vi "Read All Files In Folder.vi"(8 "error in (no error)":errorcluster, 10 "FolderPath":path, 11 "Old File Path":path) -> (0 "error out":errorcluster, 1 "File Name":string, 2 "New File Path":path, 3 "File Paths":path[](array[path]))   [LabVIEW 2020, in "DocTool.lvlib"]
uses:
  DocTool.lvlib
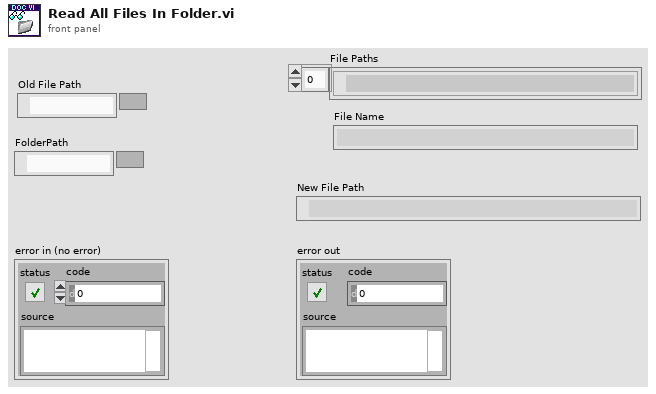
[diagram p1: front panel]
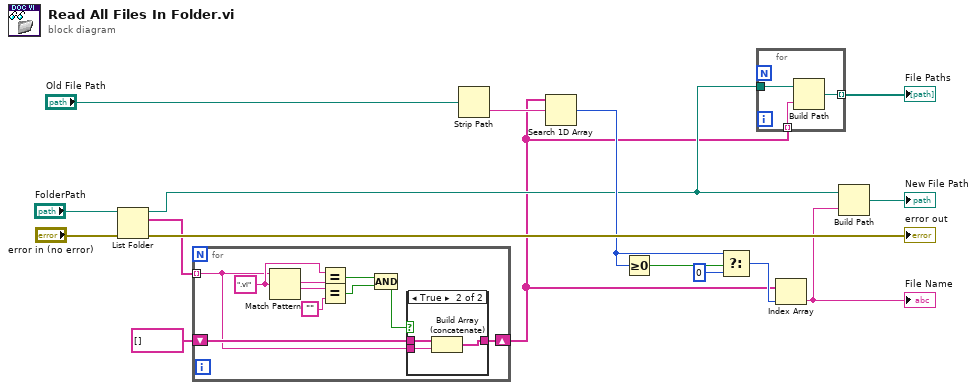
[diagram p0: block diagram]
diagram:
  n1 = List Folder(path="FolderPath", error in="error in (no error)") -> (path out=w5:path, filenames=w4:string[], error out=→"error out":errorcluster)  [unwired: 2 in, 1 out]
  n2 = for {
    tunnel: w4 -> [w20] mode=indexing
    shift-right: [w25] -> w1
    shift-left: string[] [] ("filenames") -> [w26]
    w21 = ".vi" ("string")
    n3 = Match Pattern(string=w20, regular expression=w21) -> (match substring=w22:string, after substring=w24:string)  [unwired: 1 in, 2 out]
    n4 = Equal?(x=w21, y=w22) -> (x = y?=w17:bool)
    n5 = Equal?(x=w24, y="") -> (x = y?=w18:bool)
    n6 = Compound Arithmetic op=AND(w17, w18) -> (w19:bool)
    n7 = case shown="True" w19 {
      tunnel: w26 -> [w27 w30]
      tunnel: [w27 w29] -> w25
      tunnel: w20 -> [_ w28]
      frame False {
      }
      frame True {
        n8 = Build Array (concatenate)(w30, w28) -> (w29:string[])
      }
    }
  }
  n9 = Strip Path(path="Old File Path") -> (name=w10:string)  [unwired: 1 out]
  n10 = Search 1D Array(1D array=w1, element=w10) -> (index of element=w9:i32)  [unwired: 1 in]
  n11 = Greater Or Equal To 0?(x=w9) -> (x >= 0?=w8:bool)
  n12 = Select(t=w9, s=w8, f=0) -> (s? t:f=w6:i32)
  n13 = for {
    tunnel: w5 -> [w33]
    tunnel: w1 -> [w32] mode=indexing
    tunnel: [w31] -> w3 mode=indexing
    n14 = Build Path(base path=w33, name or relative path=w32) -> (appended path=w31:path)
  }
  "File Paths" <- w3
  n15 = Index Array(array=w1, index=w6) -> (element=w13:string)
  "File Name" <- w13
  n16 = Build Path(base path=w5, name or relative path=w13) -> (appended path=→"New File Path":path)
